vi "Formula_Generater.vi"(6 "error in (no error)":errorcluster, 7 "functionInfo":T1={"time1"=0.0, "formula1"="0", "time2"=0.0, "formula2"="0", "time3"=0.0, "formula3"="0", "time4"=0.0, "formula4"="0"}, 8 "scale":dbl=1.0 format="%0.2f", 9 "offset":dbl format="%0.2p", 11 "sampling info":cluster{"Fs":dbl, "#s":dbl}={"Fs"=1000.0, "#s"=1000.0} {"Fs" format="%.2p"}) -> (4 "error out":errorcluster, 5 "waveform out":waveform(dbl))   [LabVIEW 2021]
uses:
  <vilib>/Waveform/WDTOps.llb/WDT Append Waveforms DBL.vi
  <vilib>/measure/NI_MAPro.lvlib
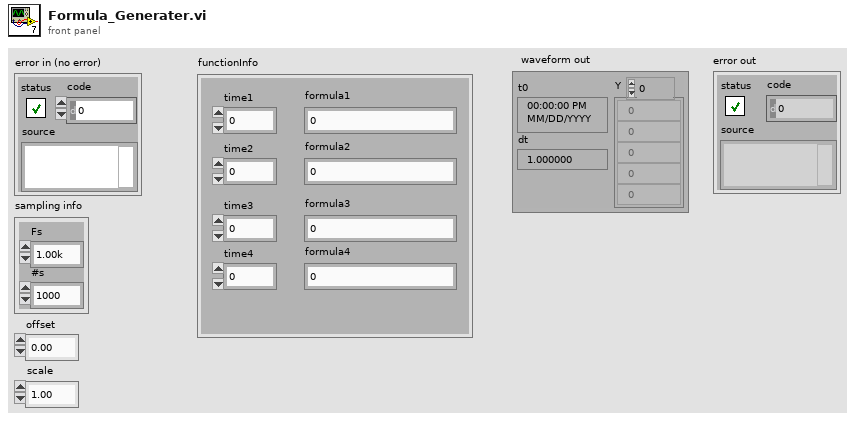
[diagram p1: front panel]
types:
  T1 = cluster{"time1":dbl, "formula1":string, "time2":dbl, "formula2":string, "time3":dbl, "formula3":string, "time4":dbl, "formula4":string}
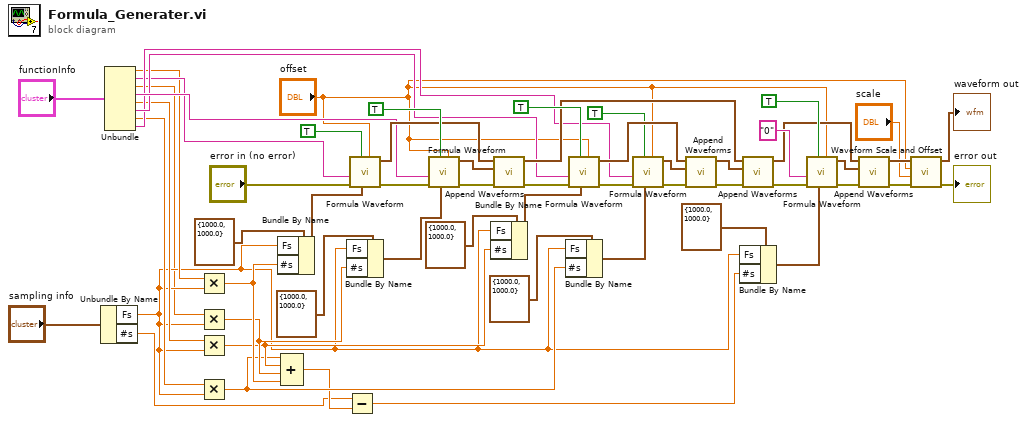
[diagram p0: block diagram]
diagram:
  n1 = Unbundle By Name("sampling info") -> ("Fs"=w2:dbl, "#s"=w8:dbl)
  n2 = Unbundle("functionInfo") -> ("time1"=w25:dbl, "formula1"=w29:string, "time2"=w1:dbl, "formula2"=w32:string, "time3"=w24:dbl, "formula3"=w31:string, "time4"=w23:dbl, "formula4"=w30:string)
  n3 = Multiply(x=w25, y=w2) -> (x*y=w13:dbl)
  n4 = Multiply(x=w1, y=w2) -> (x*y=w12:dbl)
  n5 = Multiply(x=w24, y=w2) -> (x*y=w11:dbl)
  n6 = Multiply(x=w23, y=w2) -> (x*y=w10:dbl)
  n7 = Bundle By Name(cluster=cluster{"Fs":dbl, "#s":dbl} {"Fs"=1000.0, "#s"=1000.0} ("sampling info"), "Fs"=w2, "#s"=w13) -> (w47:cluster{"Fs":dbl, "#s":dbl})
  n8 = Compound Arithmetic op=ADD(w10, w11, w12, w13) -> (w9:dbl)
  n9 = Bundle By Name(cluster=cluster{"Fs":dbl, "#s":dbl} {"Fs"=1000.0, "#s"=1000.0} ("sampling info"), "Fs"=w2, "#s"=w12) -> (w43:cluster{"Fs":dbl, "#s":dbl})
  n10 = Subtract(x=w8, y=w9) -> (x-y=w7:dbl)
  n11 = call <vilib>:"Formula Waveform.vi"("offset"="offset", "sampling info"=w47, "reset signal"=TRUE, "error in (no error)"="error in (no error)", "formula"=w29) -> ("error out"=w54:errorcluster, "signal out"=w53:waveform(dbl))  [unwired: 5 in]
  n12 = call <vilib>:"Formula Waveform.vi"("offset"="offset", "sampling info"=w43, "reset signal"=TRUE, "error in (no error)"=w54, "formula"=w32) -> ("error out"=w51:errorcluster, "signal out"=w52:waveform(dbl))  [unwired: 5 in]
  n13 = Bundle By Name(cluster=cluster{"Fs":dbl, "#s":dbl} {"Fs"=1000.0, "#s"=1000.0} ("sampling info"), "Fs"=w2, "#s"=w11) -> (w45:cluster{"Fs":dbl, "#s":dbl})
  n14 = call-poly <vilib>:"Append Waveforms.vi"("error in (no error)"=w51, "waveform B"=w52, "waveform A"=w53) -> ("error out"=w50:errorcluster, "waveform out"=w49:waveform(dbl))  [unwired: 7 in]
  n15 = Bundle By Name(cluster=cluster{"Fs":dbl, "#s":dbl} {"Fs"=1000.0, "#s"=1000.0} ("sampling info"), "Fs"=w2, "#s"=w10) -> (w26:cluster{"Fs":dbl, "#s":dbl})
  n16 = call <vilib>:"Formula Waveform.vi"("offset"="offset", "sampling info"=w45, "reset signal"=TRUE, "error in (no error)"=w50, "formula"=w31) -> ("error out"=w39:errorcluster, "signal out"=w40:waveform(dbl))  [unwired: 5 in]
  n17 = call <vilib>:"Formula Waveform.vi"("offset"="offset", "sampling info"=w26, "reset signal"=TRUE, "error in (no error)"=w39, "formula"=w30) -> ("error out"=w37:errorcluster, "signal out"=w38:waveform(dbl))  [unwired: 5 in]
  n18 = call-poly <vilib>:"Append Waveforms.vi"("error in (no error)"=w37, "waveform B"=w38, "waveform A"=w40) -> ("error out"=w35:errorcluster, "waveform out"=w34:waveform(dbl))  [unwired: 7 in]
  n19 = Bundle By Name(cluster=cluster{"Fs":dbl, "#s":dbl} {"Fs"=1000.0, "#s"=1000.0} ("sampling info"), "Fs"=w2, "#s"=w7) -> (w6:cluster{"Fs":dbl, "#s":dbl})
  n20 = call-poly <vilib>:"Append Waveforms.vi"("error in (no error)"=w35, "waveform B"=w34, "waveform A"=w49) -> ("error out"=w22:errorcluster, "waveform out"=w17:waveform(dbl))  [unwired: 7 in]
  n21 = call <vilib>:"Formula Waveform.vi"("offset"="offset", "sampling info"=w6, "reset signal"=TRUE, "error in (no error)"=w22, "formula"="0") -> ("error out"=w15:errorcluster, "signal out"=w18:waveform(dbl))  [unwired: 5 in]
  n22 = call-poly <vilib>:"Append Waveforms.vi"("error in (no error)"=w15, "waveform B"=w18, "waveform A"=w17) -> ("error out"=w14:errorcluster, "waveform out"=w16:waveform(dbl))  [unwired: 7 in]
  n23 = call <vilib>:"Waveform Scale and Offset.vi"("error in (no error)"=w14, "scale"="scale", "offset"="offset", "waveform in"=w16) -> ("error out"=→"error out":errorcluster, "waveform out"=→"waveform out":waveform(dbl))  [unwired: 6 in]
